vi "Setpoint Autostep.vi"(10 "delta(s)":dbl=1.0, 11 "Ping-pong":bool) -> (1 "Setpoint":dbl, 2 "Toggle":bool, 3 "millisecond out":u32)   [LabVIEW 2020]
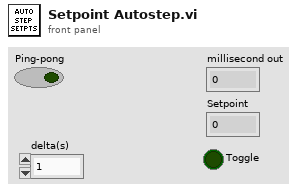
[diagram p1: front panel]
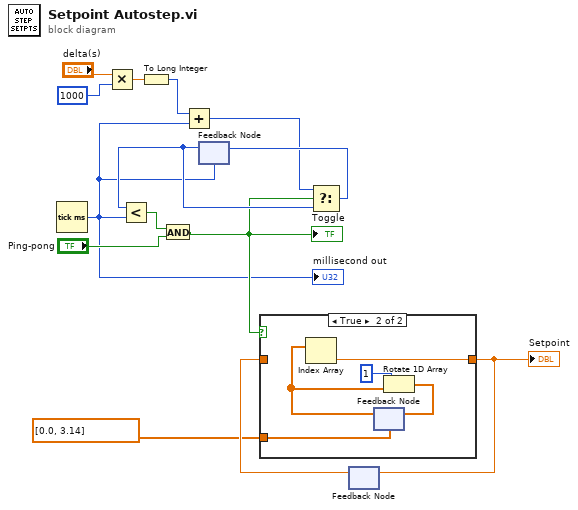
[diagram p0: block diagram]
diagram:
  n1 = Tick Count (ms)() -> (millisecond timer value=w2:u32)
  "millisecond out" <- w2
  n2 = Multiply(x="delta(s)", y=1000) -> (x*y=w5:dbl)
  n3 = To Long Integer(number=w5) -> (32bit integer=w3:i32)
  n4 = Add(x=w3, y=w2) -> (x+y=w4:u32)
  n5 = feedback #1(w2) -> (w12:u32)
  n6 = Less?(x=w12, y=w2) -> (x < y?=w14:bool)
  n7 = And(x=w14, y="Ping-pong") -> (x .and. y?=w10:bool)
  "Toggle" <- w10
  n8 = Select(t=w4, s=w10, f=w12) -> (s? t:f=w11:u32)
  n9 = feedback-in #1(w11) -> ()
  n10 = feedback #2() -> (w8:dbl)  [unwired: 1 in]
  n11 = case shown="True" w10 {
    tunnel: [w15 w17] -> w9
    tunnel: w8 -> [w15 _]
    tunnel: dbl[] [0.0, 3.14] -> [_ w16]
    frame False {
    }
    frame True {
      n12 = feedback #3(w16) -> (w18:dbl[])
      n13 = Index Array(array=w18) -> (element=w17:dbl)  [unwired: 1 in]
      n14 = Rotate 1D Array(1:w18, 2:1 ("n")) -> (0:w19:dbl[])
      n15 = feedback-in #3(w19) -> ()
    }
  }
  "Setpoint" <- w9
  n16 = feedback-in #2(w9) -> ()
